vi "Point&Path@EnableAxis__Parameter.vi"(1 "ParamterIn":string) -> (0 "ParamterOut":string)   [LabVIEW 2019]
panel:
  in  "Parameter":string(combo)
  in  "PointName":string(combo)
  in  "Confirm":bool
  # "Point&Path@EnableAxis $Point,$AXIS"
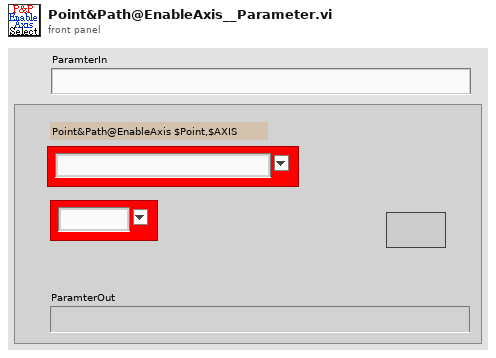
[diagram p1: front panel]
types:
  T1 = enum16{"Get", "UpdatePointS", "Init", "UpdateIndex", "GetCurrent&Index+1", "GetWithIndex", "ChkLast", "GetCurrent"}
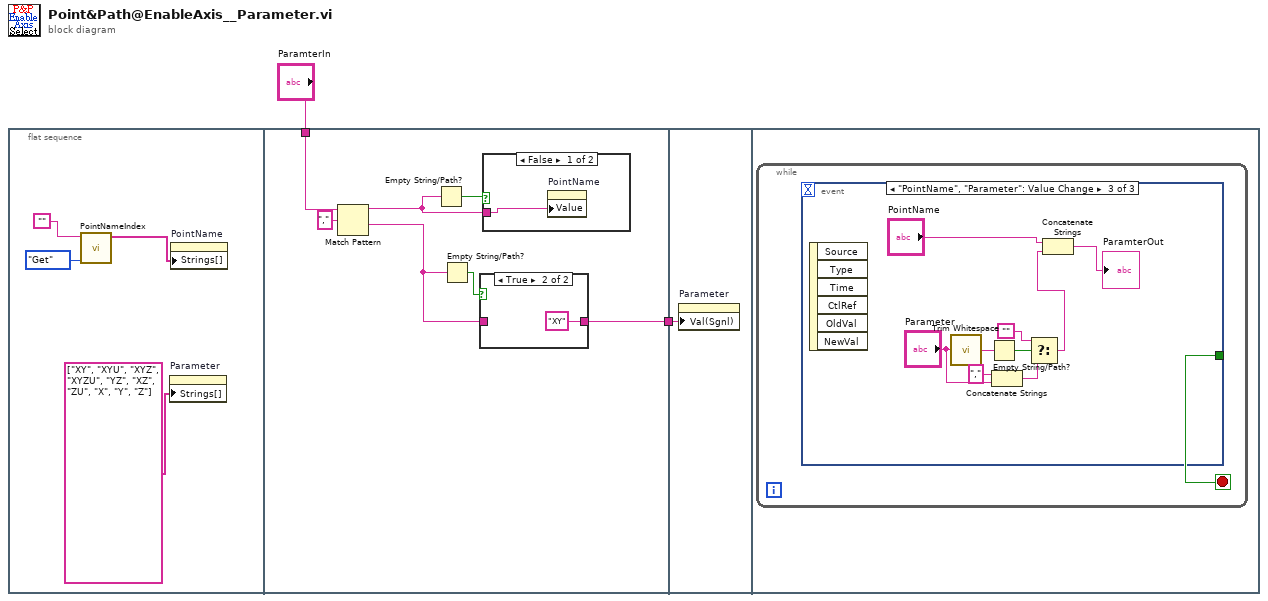
[diagram p0: block diagram]
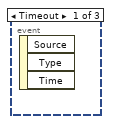
[diagram p4: hidden frame]
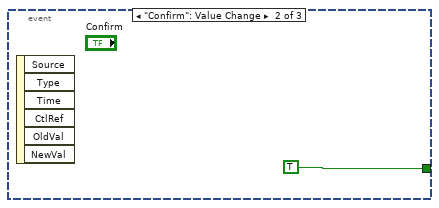
[diagram p5: hidden frame]
diagram:
  n1 = flat-sequence {
    tunnel: "ParamterIn" -> [w10]
    tunnel: [w11] -> w1
    tunnel: w1 -> [w17]
    frame #0 {
      n2 = call "PointNameIndex.vi"("OP"=T1."Get", "PointName"="") -> ("PointNameList"=w4:string[])  [unwired: 4 in, 5 out]
      n3 = property on="Parameter" class="CmbBox"("Strings[]"=string[] ["XY", "XYU", "XYZ", "XYZU", "YZ", "XZ", "ZU", "X", "Y", "Z"] ("Strings []")) -> ()  [unwired: 2 in, 2 out]
      n4 = property on="PointName" class="CmbBox"("Strings[]"=w4) -> ()  [unwired: 2 in, 2 out]
    }
    frame #1 {
      n5 = Match Pattern(string=w10, regular expression="," ("search string")) -> (before substring=w7:string, after substring=w8:string)  [unwired: 1 in, 2 out]
      n6 = Empty String/Path?(string/path=w7) -> (empty?=w13:bool)
      n7 = Empty String/Path?(string/path=w8) -> (empty?=w12:bool)
      n8 = case shown="True" w12 {
        tunnel: [w14 "XY"] -> w11
        tunnel: w8 -> [w14 _]
        frame False {
        }
        frame True {
        }
      }
      n9 = case shown="False" w13 {
        tunnel: w7 -> [w16 _]
        frame False {
          n10 = property on="PointName" class="CmbBox"("Value"=w16) -> ()  [unwired: 2 in, 2 out]
        }
        frame True {
        }
      }
    }
    frame #2 {
      n11 = property on="Parameter" class="CmbBox"("Val(Sgnl)"=w17) -> ()  [unwired: 2 in, 2 out]
    }
    frame #3 {
      n12 = while {
        stop <- w18 stop-if-true
        n13 = event shown="[2] \"PointName\", \"Parameter\": Value Change" {
          selector: _ -> [_ _ _]
          dyn-events: _ -> [_ _ _]
          timeout: _ -> [_ _ _]
          tunnel: [_ TRUE _] -> w18
          event Timeout {
            n14 = event-data() -> ()  [unwired: 1 in, 3 out]
          }
          event "Confirm": Value Change {
            n15 = event-data() -> ()  [unwired: 1 in, 6 out]
          }
          event "PointName", "Parameter": Value Change {
            n16 = event-data() -> ()  [unwired: 1 in, 6 out]
            n17 = call <vilib>:"Trim Whitespace.vi"("string"="Parameter") -> ("trimmed string"=w23:string)  [unwired: 1 in]
            n18 = Empty String/Path?(string/path=w23) -> (empty?=w24:bool)
            n19 = Concatenate Strings("," ("string"), "Parameter") -> (w26:string)
            n20 = Select(t="", s=w24, f=w26) -> (s? t:f=w21:string)
            n21 = Concatenate Strings("PointName", w21) -> (→"ParamterOut":string)
          }
        }
      }
    }
  }
